vi "Confirm IP address.vi"(8 "error in":errorcluster) -> (0 "error out":errorcluster)   [LabVIEW 2024, in "Session Scanner.lvlib"]
doc: "Retrieves IP address or Hostname from input data in case the user only knows one of these fields"
uses:
  Session Scanner.lvlib
  Support/General Type Defs/Global Data.vi
  Support/General Type Defs/General Type Definitions.lvlib
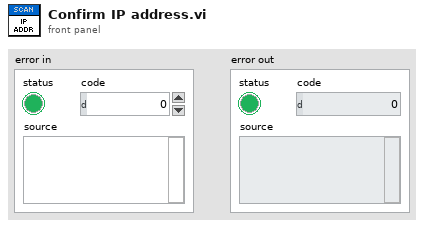
[diagram p1: front panel]
types:
  T1 = typedef "General Type Definitions.lvlib/Device Data.ctl" = cluster{"OS":T2, "User":string, "Password":string, "Hostname":string, "IP Address":string}
  T2 = typedef "General Type Definitions.lvlib/Device OS.ctl" = enum16{"Windows", "Linux"}
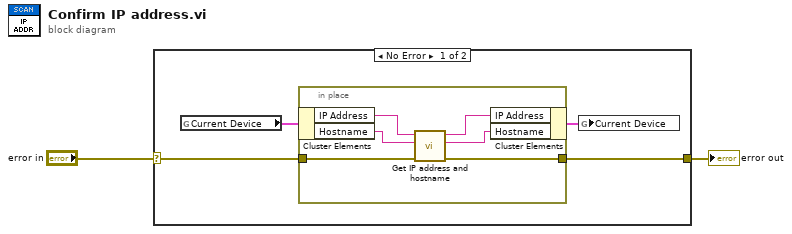
[diagram p0: block diagram]
diagram:
  n1 = case shown="No Error" "error in" {
    selector: "error in" -> [w5 w13]
    tunnel: [w6 w13] -> w2
    frame No Error {
      n2 = global read "Global Data.vi" "Current Device"() -> (w4:T1)
      n3 = in-place {
        in-place-border: [w12] -> w6
        in-place-border: w5 -> [w11]
        n4 = in-place-cluster #1(w4) -> ("IP Address"=w9:string, "Hostname"=w10:string)
        n5 = call "Get IP address and hostname.vi"("error in (no error)"=w11, "Hostname In"=w10, "IP Address In"=w9) -> ("error out"=w12:errorcluster, "Found Hostname"=w7:string, "Found IP"=w8:string)  [unwired: 6 in]
        n6 = in-place-cluster #1("IP Address"=w8, "Hostname"=w7) -> (w3:T1)
      }
      n7 = global write "Global Data.vi" "Current Device"(w3) -> ()
    }
    frame Error {
    }
  }
  "error out" <- w2
